vi "ErrorViewer.Start.vi"(5 "Autoshutdown? (T)":bool=TRUE, 8 "error in (no error)":errorcluster, 11 "NewTemplate in":refnum<class "ErrorViewer.lvclass">) -> (0 "error out":errorcluster, 1 "StartupHandshake out":refnum<class "ModuleStartup.lvclass">, 2 "_TemplateModule":cluster{"Broadcasts":T1, "Broadcasts":T2}, 3 "NewTemplate out":refnum<class "ErrorViewer.lvclass">)   [LabVIEW 2024, in "ErrorViewer.lvclass"]
uses:
  ErrorViewer.lvclass
  C:/Git/JA/JQMH/RQMHCore/ModuleCore/Module.lvclass
  RQMHCore/Startup/ModuleStartup.lvclass
  ErrorViewer.lvclass/ErrorViewer.ctl
  RQMHCore/ModuleCore/Module.lvclass
  Stopped.ctl
  Broadcast Events--cluster.ctl
  RQMHCore/Shared/Died.ctl
  RQMHCore/Shared/ModuleShared.lvlib
  RQMHCore/ModuleCore/StandardBroadcasts.ctl
  RQMHCore/ModuleCore/Started.ctl
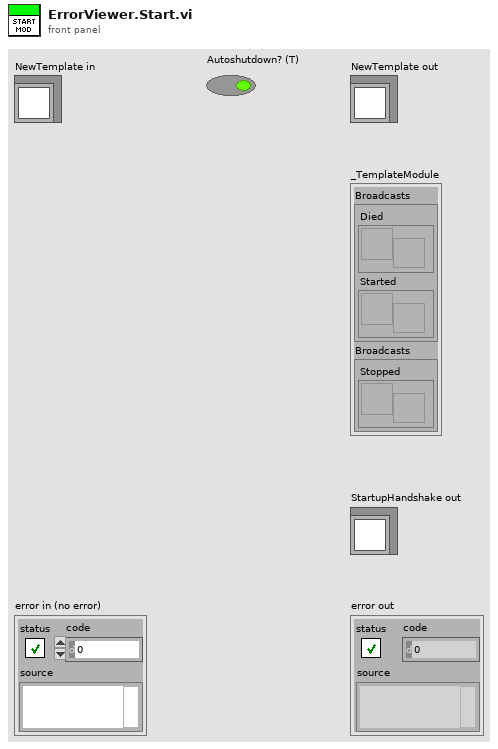
[diagram p1: front panel]
types:
  T1 = typedef "Module.lvclass/StandardBroadcasts.ctl" = cluster{"Died":refnum<user-event>, "Started":refnum<user-event>}
  T2 = typedef "ErrorViewer.lvclass/Broadcast Events--cluster.ctl" = cluster{"Stopped":refnum<user-event>}
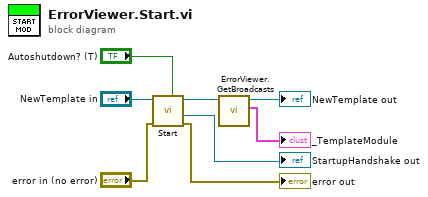
[diagram p0: block diagram]
diagram:
  n1 = call "Start.vi"("Autoshutdown? (T)"="Autoshutdown? (T)", "error in (no error)"="error in (no error)", "JQMHCore in"="NewTemplate in") -> ("error out"=→"error out":errorcluster, "StartupHandshake out"=→"StartupHandshake out":refnum<class "ModuleStartup.lvclass">, "JQMHCore out"=w4:refnum<class "ErrorViewer.lvclass">)  [unwired: 6 in]
  n2 = call "ErrorViewer.GetBroadcasts.vi"("NewTemplate in"=w4) -> ("SingleLoopTemplate"=→"_TemplateModule":cluster{"Broadcasts":T1, "Broadcasts":T2}, "NewTemplate out"=→"NewTemplate out":refnum<class "ErrorViewer.lvclass">)  [unwired: 9 in]
